vi "LM Two Gaussians and gradient.vi"(3 "output control":T1, 4 "data":variant, 5 "X":dbl[](array[numeric]), 6 "a":dbl[](array[numeric])) -> (0 "error out":errorcluster, 1 "f'(X,a)":dbl[][](array[numeric]), 2 "f(X,a)":dbl[](array[numeric]))   [LabVIEW 2021, in "Fits.lvlib"]
doc: "This template is the starting point for creating a model function to be passed to the Nonlinear Curve Fit.vi."
uses:
  Fits.lvlib
  <vilib>/gmath/NumericalOptimization/LM_output select.ctl
  D-Only Fixed Parameters.ctl
  <vilib>/gmath/NI_Gmath.lvlib
panel:
  # "Parameters:\n\namplitude 1: A1\ncenter 1: t1\nSDV 1: s1\nAmplitude 2: A2\ncenter 2: t2\nSDV 2: s2"
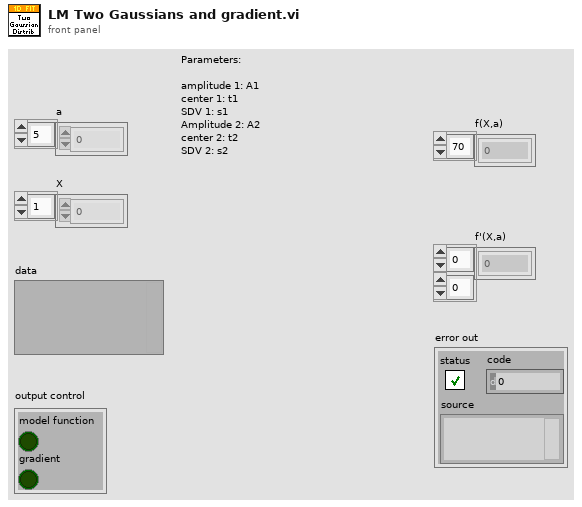
[diagram p1: front panel]
types:
  T1 = typedef "NI_Gmath.lvlib/LM_output select.ctl" = cluster{"model function":bool, "gradient":bool}
  T2 = typedef "Fits.lvlib/D-Only Fixed Parameters.ctl" = cluster{"Fix D-only Peak Location":bool, "Peak Location":dbl, "Fix D-only Peak FWHM":bool, "Peak FWHM":dbl}
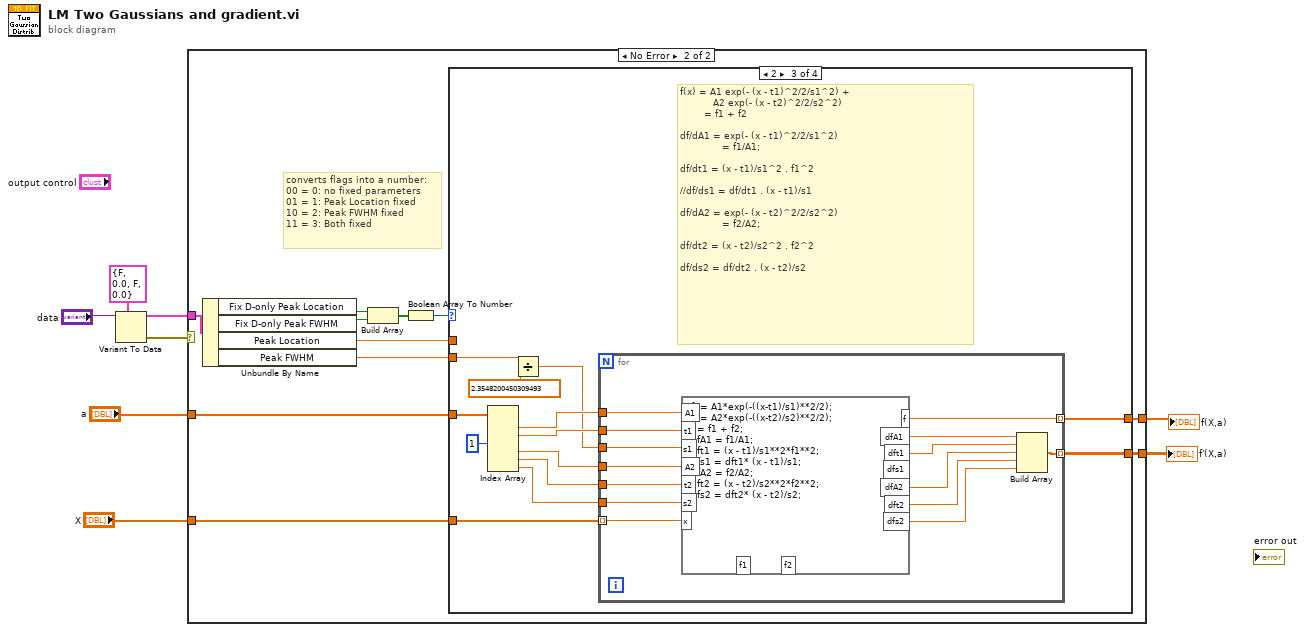
[diagram p0: block diagram]
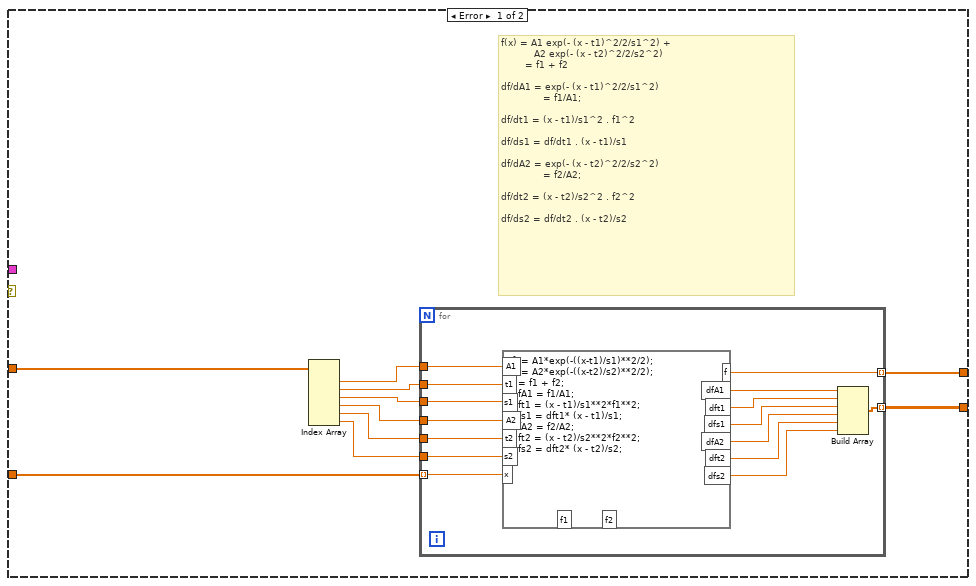
[diagram p2: hidden frame]
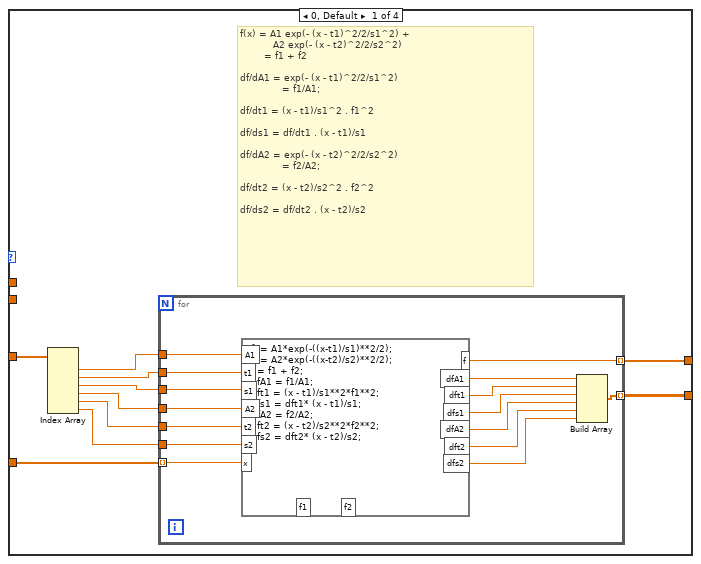
[diagram p3: hidden frame]
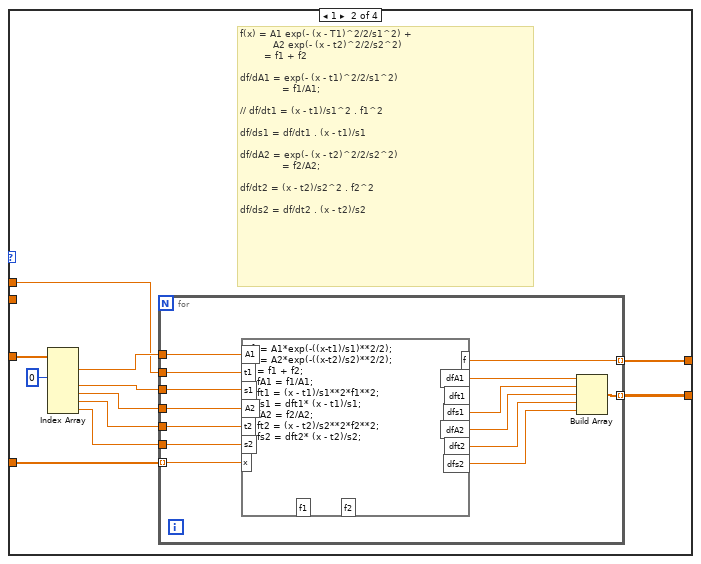
[diagram p4: hidden frame]
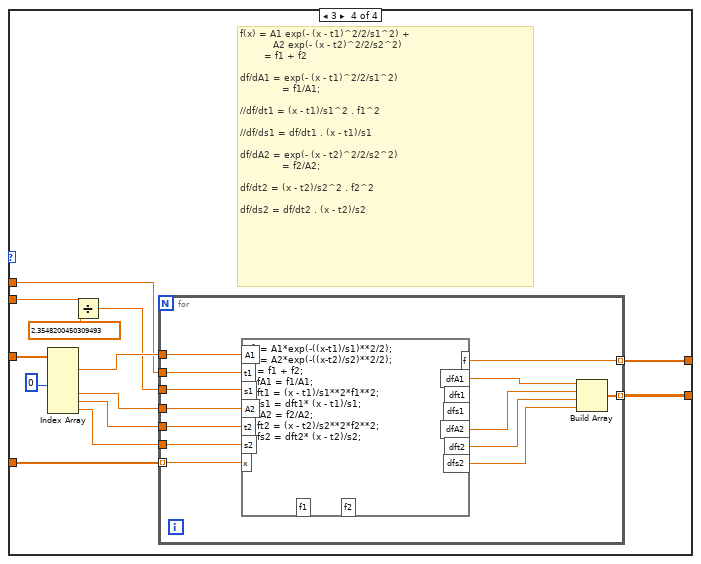
[diagram p5: hidden frame]
diagram:
  n1 = Variant To Data(type=T2 {"Fix D-only Peak Location"=FALSE, "Peak Location"=0.0, "Fix D-only Peak FWHM"=FALSE, "Peak FWHM"=0.0} ("Fixed Parameters"), Variant="data") -> (data=w1:T2, error out=w2:errorcluster)  [unwired: 1 in]
  n2 = case shown="No Error" w2 {
    tunnel: "a" -> [w18 w44]
    tunnel: "X" -> [w17 w43]
    tunnel: [w16 w42] -> w6
    tunnel: [w15 w41] -> w5
    tunnel: w1 -> [_ w40]
    frame Error {
      # "f(x) = A1 exp(- (x - t1)^2/2/s1^2) +\n           A2 exp(- (x - t2)^2/2/s2^2)\n        = f1 + f2\n\ndf/dA1 = exp(- (x - t1)^2/2/s1^2)\n              = f1/A1;\n\ndf/dt1 = (x - t1)/s1^2 . f1^2\n\ndf/ds1 = df/dt1 . (x - t1)/s1                     \n\ndf/dA2 = exp(- (x - t2)^2/2/s2^2)\n              = f2/A2;\n\ndf/dt2 = (x - t2)/s2^2 . f2^2\n\ndf/ds2 = df/dt2 . (x - t2)/s2"
      n3 = Index Array(array=w18) -> (element #1=w14:dbl, element #2=w13:dbl, element #3=w12:dbl, element #4=w11:dbl, element #5=w10:dbl, element #6=w9:dbl)  [unwired: 6 in]
      n4 = for {
        tunnel: w17 -> [w33] mode=indexing
        tunnel: [w31] -> w16 mode=indexing
        tunnel: [w30] -> w15 mode=indexing
        tunnel: w14 -> [w29]
        tunnel: w13 -> [w28]
        tunnel: w12 -> [w27]
        tunnel: w11 -> [w26]
        tunnel: w10 -> [w25]
        tunnel: w9 -> [w24]
        n5 = formula code="f1= A1*exp(-((x-t1)/s1)**2/2);\nf2= A2*exp(-((x-t2)/s2)**2/2);\nf = f1 + f2;\ndfA1 = f1/A1;\ndft1 = (x - t1)/s1**2*f1**2;\ndfs1 = dft1* (x - t1)/s1;\ndfA2 = f2/A2;\ndft2 = (x - t2)/s2**2*f2**2;\ndfs2 = dft2* (x - t2)/s2;"("A1"=w29, "t1"=w28, "s1"=w27, "x"=w33, "A2"=w26, "t2"=w25, "s2"=w24) -> ("f"=w31:dbl, "dfA1"=w32:dbl, "dft1"=w23:dbl, "dfs1"=w22:dbl, "dfA2"=w21:dbl, "dft2"=w20:dbl, "dfs2"=w19:dbl)  [unwired: 2 out]
        n6 = Build Array(w32, w23, w22, w21, w20, w19) -> (w30:dbl[])
      }
    }
    frame No Error {
      # "converts flags into a number:\n00 = 0: no fixed parameters\n01 = 1: Peak Location fixed\n10 = 2: Peak FWHM fixed\n11 = 3: Both fixed"
      n7 = Unbundle By Name(w40) -> ("Fix D-only Peak Location"=w39:bool, "Fix D-only Peak FWHM"=w38:bool, "Peak Location"=w35:dbl, "Peak FWHM"=w34:dbl)
      n8 = Build Array(w39, w38) -> (w37:bool[])
      n9 = Boolean Array To Number(Boolean array=w37) -> (number=w36:u32)
      n10 = case shown="2" w36 {
        tunnel: w44 -> [w54 w80 w107 w134]
        tunnel: w43 -> [w53 w79 w106 w133]
        tunnel: [w52 w78 w105 w132] -> w42
        tunnel: [w51 w77 w104 w131] -> w41
        tunnel: w35 -> [_ w71 _ w123]
        tunnel: w34 -> [_ _ w98 w126]
        frame 0, Default {
          # "f(x) = A1 exp(- (x - t1)^2/2/s1^2) +\n           A2 exp(- (x - t2)^2/2/s2^2)\n        = f1 + f2\n\ndf/dA1 = exp(- (x - t1)^2/2/s1^2)\n              = f1/A1;\n\ndf/dt1 = (x - t1)/s1^2 . f1^2\n\ndf/ds1 = df/dt1 . (x - t1)/s1                     \n\ndf/dA2 = exp(- (x - t2)^2/2/s2^2)\n              = f2/A2;\n\ndf/dt2 = (x - t2)/s2^2 . f2^2\n\ndf/ds2 = df/dt2 . (x - t2)/s2"
          n11 = Index Array(array=w54) -> (element #1=w50:dbl, element #2=w49:dbl, element #3=w48:dbl, element #4=w47:dbl, element #5=w46:dbl, element #6=w45:dbl)  [unwired: 6 in]
          n12 = for {
            tunnel: w53 -> [w69] mode=indexing
            tunnel: [w67] -> w52 mode=indexing
            tunnel: [w66] -> w51 mode=indexing
            tunnel: w50 -> [w65]
            tunnel: w49 -> [w64]
            tunnel: w48 -> [w63]
            tunnel: w47 -> [w62]
            tunnel: w46 -> [w61]
            tunnel: w45 -> [w60]
            n13 = formula code="f1= A1*exp(-((x-t1)/s1)**2/2);\nf2= A2*exp(-((x-t2)/s2)**2/2);\nf = f1 + f2;\ndfA1 = f1/A1;\ndft1 = (x - t1)/s1**2*f1**2;\ndfs1 = dft1* (x - t1)/s1;\ndfA2 = f2/A2;\ndft2 = (x - t2)/s2**2*f2**2;\ndfs2 = dft2* (x - t2)/s2;"("A1"=w65, "t1"=w64, "s1"=w63, "x"=w69, "A2"=w62, "t2"=w61, "s2"=w60) -> ("f"=w67:dbl, "dfA1"=w68:dbl, "dft1"=w59:dbl, "dfs1"=w58:dbl, "dfA2"=w57:dbl, "dft2"=w56:dbl, "dfs2"=w55:dbl)  [unwired: 2 out]
            n14 = Build Array(w68, w59, w58, w57, w56, w55) -> (w66:dbl[])
          }
        }
        frame 1 {
          # "f(x) = A1 exp(- (x - T1)^2/2/s1^2) +\n           A2 exp(- (x - t2)^2/2/s2^2)\n        = f1 + f2\n\ndf/dA1 = exp(- (x - t1)^2/2/s1^2)\n              = f1/A1;\n\n// df/dt1 = (x - t1)/s1^2 . f1^2\n\ndf/ds1 = df/dt1 . (x - t1)/s1                     \n\ndf/dA2 = exp(- (x - t2)^2/2/s2^2)\n              = f2/A2;\n\ndf/dt2 = (x - t2)/s2^2 . f2^2\n\ndf/ds2 = df/dt2 . (x - t2)/s2"
          n15 = Index Array(array=w80, index #2=0 ("index")) -> (element #1=w76:dbl, element #3=w75:dbl, element #4=w74:dbl, element #5=w73:dbl, element #6=w72:dbl)  [unwired: 5 in, 1 out]
          n16 = for {
            tunnel: w79 -> [w94] mode=indexing
            tunnel: [w92] -> w78 mode=indexing
            tunnel: [w91] -> w77 mode=indexing
            tunnel: w76 -> [w90]
            tunnel: w71 -> [w89]
            tunnel: w75 -> [w88]
            tunnel: w74 -> [w87]
            tunnel: w73 -> [w86]
            tunnel: w72 -> [w85]
            n17 = formula code="f1= A1*exp(-((x-t1)/s1)**2/2);\nf2= A2*exp(-((x-t2)/s2)**2/2);\nf = f1 + f2;\ndfA1 = f1/A1;\ndft1 = (x - t1)/s1**2*f1**2;\ndfs1 = dft1* (x - t1)/s1;\ndfA2 = f2/A2;\ndft2 = (x - t2)/s2**2*f2**2;\ndfs2 = dft2* (x - t2)/s2;"("A1"=w90, "t1"=w89, "s1"=w88, "x"=w94, "A2"=w87, "t2"=w86, "s2"=w85) -> ("f"=w92:dbl, "dfA1"=w93:dbl, "dfs1"=w84:dbl, "dfA2"=w83:dbl, "dft2"=w82:dbl, "dfs2"=w81:dbl)  [unwired: 3 out]
            n18 = Build Array(w93, w84, w83, w82, w81) -> (w91:dbl[])
          }
        }
        frame 2 {
          # "f(x) = A1 exp(- (x - t1)^2/2/s1^2) +\n           A2 exp(- (x - t2)^2/2/s2^2)\n        = f1 + f2\n\ndf/dA1 = exp(- (x - t1)^2/2/s1^2)\n              = f1/A1;\n\ndf/dt1 = (x - t1)/s1^2 . f1^2\n\n//df/ds1 = df/dt1 . (x - t1)/s1                     \n\ndf/dA2 = exp(- (x - t2)^2/2/s2^2)\n              = f2/A2;\n\ndf/dt2 = (x - t2)/s2^2 . f2^2\n\ndf/ds2 = df/dt2 . (x - t2)/s2"
          n19 = Index Array(array=w107, index #3=1 ("index")) -> (element #1=w103:dbl, element #2=w102:dbl, element #4=w101:dbl, element #5=w100:dbl, element #6=w99:dbl)  [unwired: 5 in, 1 out]
          n20 = Divide(x=w98, y=2.3548200450309493) -> (x/y=w96:dbl)
          n21 = for {
            tunnel: w106 -> [w121] mode=indexing
            tunnel: [w119] -> w105 mode=indexing
            tunnel: [w118] -> w104 mode=indexing
            tunnel: w103 -> [w117]
            tunnel: w102 -> [w116]
            tunnel: w96 -> [w115]
            tunnel: w101 -> [w114]
            tunnel: w100 -> [w113]
            tunnel: w99 -> [w112]
            n22 = formula code="f1= A1*exp(-((x-t1)/s1)**2/2);\nf2= A2*exp(-((x-t2)/s2)**2/2);\nf = f1 + f2;\ndfA1 = f1/A1;\ndft1 = (x - t1)/s1**2*f1**2;\ndfs1 = dft1* (x - t1)/s1;\ndfA2 = f2/A2;\ndft2 = (x - t2)/s2**2*f2**2;\ndfs2 = dft2* (x - t2)/s2;"("A1"=w117, "t1"=w116, "s1"=w115, "x"=w121, "A2"=w114, "t2"=w113, "s2"=w112) -> ("f"=w119:dbl, "dfA1"=w120:dbl, "dft1"=w111:dbl, "dfA2"=w110:dbl, "dft2"=w109:dbl, "dfs2"=w108:dbl)  [unwired: 3 out]
            n23 = Build Array(w120, w111, w110, w109, w108) -> (w118:dbl[])
          }
        }
        frame 3 {
          # "f(x) = A1 exp(- (x - t1)^2/2/s1^2) +\n           A2 exp(- (x - t2)^2/2/s2^2)\n        = f1 + f2\n\ndf/dA1 = exp(- (x - t1)^2/2/s1^2)\n              = f1/A1;\n\n//df/dt1 = (x - t1)/s1^2 . f1^2\n\n//df/ds1 = df/dt1 . (x - t1)/s1                     \n\ndf/dA2 = exp(- (x - t2)^2/2/s2^2)\n              = f2/A2;\n\ndf/dt2 = (x - t2)/s2^2 . f2^2\n\ndf/ds2 = df/dt2 . (x - t2)/s2"
          n24 = Index Array(array=w134, index #3=0 ("index")) -> (element #1=w130:dbl, element #4=w129:dbl, element #5=w128:dbl, element #6=w127:dbl)  [unwired: 5 in, 2 out]
          n25 = Divide(x=w126, y=2.3548200450309493) -> (x/y=w124:dbl)
          n26 = for {
            tunnel: w133 -> [w147] mode=indexing
            tunnel: [w145] -> w132 mode=indexing
            tunnel: [w144] -> w131 mode=indexing
            tunnel: w130 -> [w143]
            tunnel: w123 -> [w142]
            tunnel: w124 -> [w141]
            tunnel: w129 -> [w140]
            tunnel: w128 -> [w139]
            tunnel: w127 -> [w138]
            n27 = formula code="f1= A1*exp(-((x-t1)/s1)**2/2);\nf2= A2*exp(-((x-t2)/s2)**2/2);\nf = f1 + f2;\ndfA1 = f1/A1;\ndft1 = (x - t1)/s1**2*f1**2;\ndfs1 = dft1* (x - t1)/s1;\ndfA2 = f2/A2;\ndft2 = (x - t2)/s2**2*f2**2;\ndfs2 = dft2* (x - t2)/s2;"("A1"=w143, "t1"=w142, "s1"=w141, "x"=w147, "A2"=w140, "t2"=w139, "s2"=w138) -> ("f"=w145:dbl, "dfA1"=w146:dbl, "dfA2"=w137:dbl, "dft2"=w136:dbl, "dfs2"=w135:dbl)  [unwired: 4 out]
            n28 = Build Array(w146, w137, w136, w135) -> (w144:dbl[])
          }
        }
      }
    }
  }
  "f(X,a)" <- w6
  "f'(X,a)" <- w5
